vi "cheby6.vi"(1 "I":dbl, 2 "Coefs":dbl[](array[numeric]), 3 "RU/L":dbl[](array[numeric]), 4 "LIX":dbl) -> (0 "T":dbl)   [LabVIEW 2023]
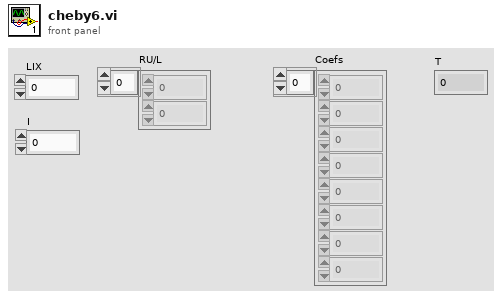
[diagram p1: front panel]
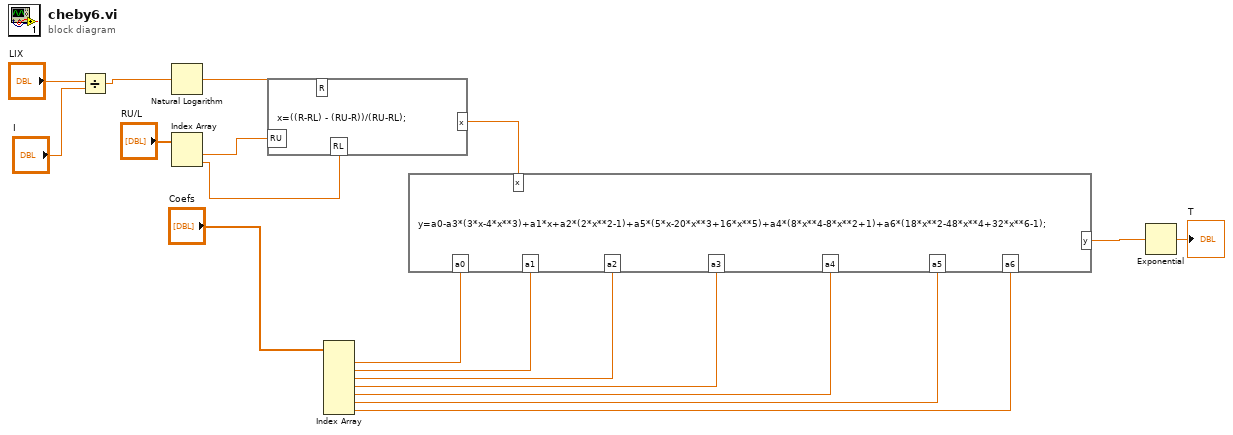
[diagram p0: block diagram]
diagram:
  n1 = Divide(x="LIX", y="I") -> (x/y=w6:dbl)
  n2 = Natural Logarithm(1:w6) -> (0:w18:dbl)
  n3 = Index Array(array="RU/L") -> (element #1=w12:dbl, element #2=w11:dbl)  [unwired: 2 in]
  n4 = formula code="x=((R-RL) - (RU-R))/(RU-RL);"("R"=w18, "RU"=w12, "RL"=w11) -> ("x"=w17:dbl)
  n5 = Index Array(array="Coefs") -> (element #1=w5:dbl, element #2=w4:dbl, element #3=w3:dbl, element #4=w2:dbl, element #5=w1:dbl, element #6=w10:dbl, element #7=w9:dbl)  [unwired: 7 in]
  n6 = formula code="y=a0-a3*(3*x-4*x**3)+a1*x+a2*(2*x**2-1)+a5*(5*x-20*x**3+16*x**5)+a4*(8*x**4-8*x**2+1)+a6*(18*x**2-48*x**4+32*x**6-1);"("x"=w17, "a0"=w5, "a3"=w2, "a1"=w4, "a2"=w3, "a4"=w1, "a5"=w10, "a6"=w9) -> ("y"=w16:dbl)
  n7 = Exponential(1:w16) -> (0:→"T":dbl)
